vi "Send positions to motor.vi"(6 "current code":string, 7 "enabled codes":string, 8 "error in (no error)":errorcluster, 11 "Motor in":refnum<class "Motor.lvclass">) -> (0 "error out":errorcluster, 3 "Motor out":refnum<class "Motor.lvclass">)   [LabVIEW 2018, in "Motor.lvclass"]
uses:
  Motor.lvclass
  Motor.lvclass/Motor.ctl
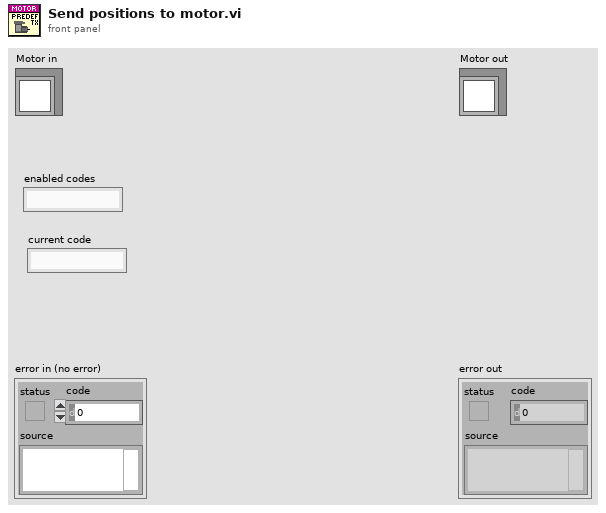
[diagram p1: front panel]
types:
  T1 = cluster{"mode":string, "condition":string, "position":string, "pos_name":string, "pos_id":string}
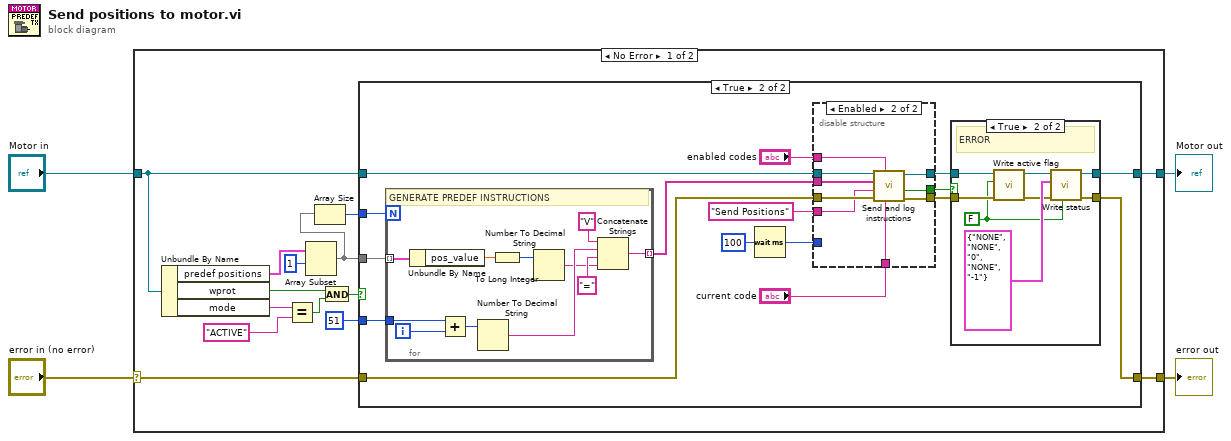
[diagram p0: block diagram]
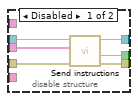
[diagram p3: hidden frame]
diagram:
  n1 = case shown="No Error" "error in (no error)" {
    selector: "error in (no error)" -> [w7 w73]
    tunnel: [w6 w73] -> w3
    tunnel: [w5 w74] -> w1
    tunnel: "Motor in" -> [w13 w74]
    frame No Error {
      n2 = Unbundle By Name(w13) -> ("predef positions"=w12:cluster{"pos_name":string, "pos_value":dbl}[], "wprot"=w17:bool, "mode"=w14:string)
      n3 = Equal?(x=w14, y="ACTIVE" ("x")) -> (x = y?=w18:bool)
      n4 = Array Subset(array=w12, index=1) -> (w9:cluster{"pos_name":string, "pos_value":dbl}[])  [unwired: 1 in]
      n5 = Array Size(array=w9) -> (size(s)=w10:i32)
      n6 = And(x=w17, y=w18) -> (x .and. y?=w16:bool)
      n7 = case shown="True" w16 {
        tunnel: w10 -> [_ w36]
        tunnel: w13 -> [w19 w33]
        tunnel: w9 -> [_ w35]
        tunnel: 51 ("x") -> [_ w34]
        tunnel: w7 -> [w20 w31]
        tunnel: [w20 w27] -> w6
        tunnel: [w19 w26] -> w5
        frame False {
        }
        frame True {
          n8 = for {
            N: w36 -> [_]
            tunnel: w35 -> [w72] mode=indexing
            tunnel: w34 -> [w68]
            tunnel: [w62] -> w32 mode=indexing
            i -> [w69]
            # "GENERATE PREDEF INSTRUCTIONS"
            n9 = Unbundle By Name(w72) -> ("pos_value"=w71:dbl)
            n10 = Add(x=w68, y=w69) -> (x+y=w67:i32)
            n11 = Number To Decimal String(number=w67) -> (decimal integer string=w65:string)  [unwired: 1 in]
            n12 = To Long Integer(number=w71) -> (32bit integer=w70:i32)
            n13 = Number To Decimal String(number=w70) -> (decimal integer string=w63:string)  [unwired: 1 in]
            n14 = Concatenate Strings("V", w65, "=", w63) -> (w62:string)
          }
          n15 = Wait (ms)(milliseconds to wait=u32 100) -> (millisecond timer value=w23:u32)
          n16 = disable-structure shown="Enabled" {
            disable-tunnel: w33 -> [w42 w51]
            disable-tunnel: w32 -> [w41 w46]
            disable-tunnel: w31 -> [w40 w49]
            disable-tunnel: [w39 w47] -> w30
            disable-tunnel: [w38 w50] -> w29
            disable-tunnel: [w37 w48] -> w28
            disable-tunnel: "current code" -> [_ w45]
            disable-tunnel: "enabled codes" -> [_ w44]
            disable-tunnel: w23 -> [_ _]
            disable-tunnel: "Send Positions" ("prefix") -> [_ w43]
            frame Disabled {
              n17 = call-dynamic "Send instructions.vi"("error in (no error)"=w40, "instructions"=w41, "Motor in"=w42) -> ("error out"=w37:errorcluster, "error"=w39:bool, "Motor out"=w38:refnum<class "Motor.lvclass">)  [unwired: 4 in, 2 out]
            }
            frame Enabled {
              n18 = call-dynamic "Send and log instructions.vi"("current code"=w45, "enabled codes"=w44, "error in (no error)"=w49, "prefix"=w43, "instructions"=w46, "Motor in"=w51) -> ("error out"=w48:errorcluster, "error"=w47:bool, "Motor out"=w50:refnum<class "Motor.lvclass">)  [unwired: 1 in, 2 out]
            }
          }
          n19 = case shown="True" w30 {
            tunnel: w29 -> [w53 w58]
            tunnel: w28 -> [w52 w55]
            tunnel: [w52 w60] -> w27
            tunnel: [w53 w59] -> w26
            frame False {
            }
            frame True {
              w54 = FALSE ("hold if empty")
              # "ERROR"
              n20 = call-dynamic "Write active flag.vi"("error in (no error)"=w55, "active"=w54, "Motor in"=w58) -> ("error out"=w56:errorcluster, "Motor out"=w57:refnum<class "Motor.lvclass">)  [unwired: 7 in]
              n21 = call-dynamic "Write status.vi"("hold if empty"=w54, "error in (no error)"=w56, "status"=T1 {"mode"="NONE", "condition"="NONE", "position"="0", "pos_name"="NONE", "pos_id"="-1"}, "Motor in"=w57) -> ("error out"=w60:errorcluster, "Motor out"=w59:refnum<class "Motor.lvclass">)  [unwired: 6 in]
            }
          }
        }
      }
    }
    frame Error {
    }
  }
  "error out" <- w3
  "Motor out" <- w1
